vi "Get Time Zone.vi"(0 "GMaps API in":refnum<class "GMaps API.lvclass">, 5 "error in (no error)":errorcluster) -> (14 "GMaps API out":refnum<class "GMaps API.lvclass">, 15 "Time Zone":T1, 19 "error out":errorcluster)   [LabVIEW 2016, in "GMaps API.lvclass"]
doc: "Gets offset data for location on the surface of the earth."
uses:
  GMaps API.lvclass
  GMaps API.lvclass/GMaps API.ctl
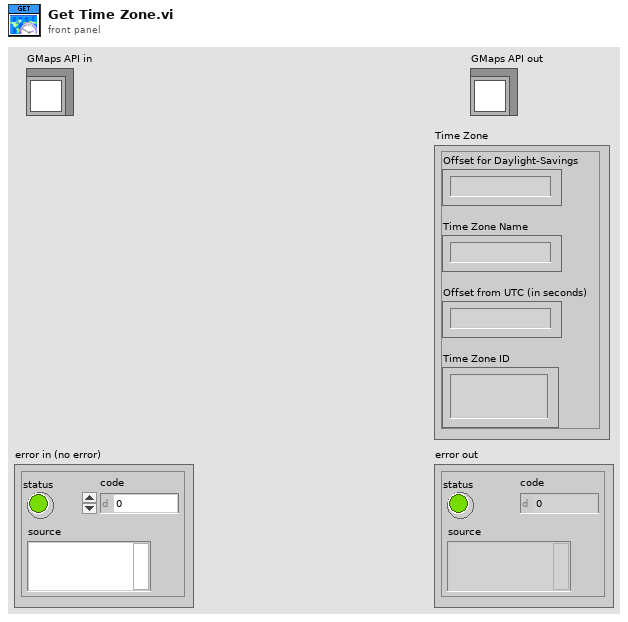
[diagram p1: front panel]
types:
  T1 = cluster{"Offset for Daylight-Savings":string, "Offset from UTC (in seconds)":string, "Time Zone Name":string, "Time Zone ID":string}
  T2 = cluster{"Time Zone ID":string, "Time Zone Name":string, "Offset for Daylight-Savings":string, "Offset from UTC (in seconds)":string}
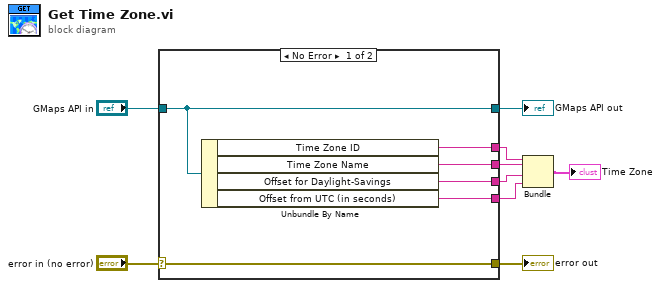
[diagram p0: block diagram]
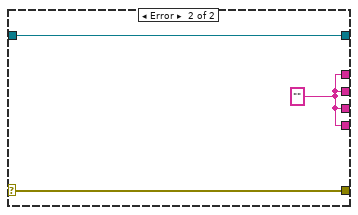
[diagram p2: hidden frame]
diagram:
  n1 = case shown="No Error" "error in (no error)" {
    selector: "error in (no error)" -> [w15 w18]
    tunnel: [w15 w18] -> w8
    tunnel: [w14 w17] -> w6
    tunnel: "GMaps API in" -> [w14 w17]
    tunnel: [w13 w16] -> w5
    tunnel: [w12 w16] -> w4
    tunnel: [w11 w16] -> w3
    tunnel: [w10 w16] -> w2
    frame No Error {
      n2 = Unbundle By Name(w14) -> ("Time Zone ID"=w13:string, "Time Zone Name"=w12:string, "Offset for Daylight-Savings"=w11:string, "Offset from UTC (in seconds)"=w10:string)
    }
    frame Error {
      w16 = ""
    }
  }
  "error out" <- w8
  "GMaps API out" <- w6
  n3 = Bundle("Time Zone ID"=w5, "Time Zone Name"=w4, "Offset for Daylight-Savings"=w3, "Offset from UTC (in seconds)"=w2) -> (→"Time Zone":T2)  [unwired: 1 in]
